vi "Shutter Control.vi"(8 "Laser Shutter":T1(radio)=enum."Off", 9 "error in":errorcluster, 11 "Camera Shutter":bool) -> ()   [LabVIEW 2014]
uses:
  Shutter SubVis/Global Shutter Variables - SubVI.vi
panel:
  out "error out":errorcluster
  out "Status":bool
  out "Current Wheel Position":string
  in  "Wheel Speed":u8=1 min=1 max=7 step=1
  in  "stop":bool
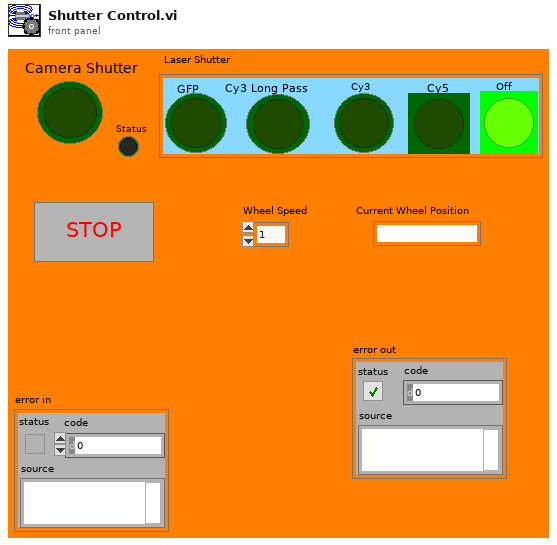
[diagram p1: front panel]
types:
  T1 = enum32{"No Selection", "GFP", "Cy3 Long Pass", "Cy3", "Cy5", "Off"}
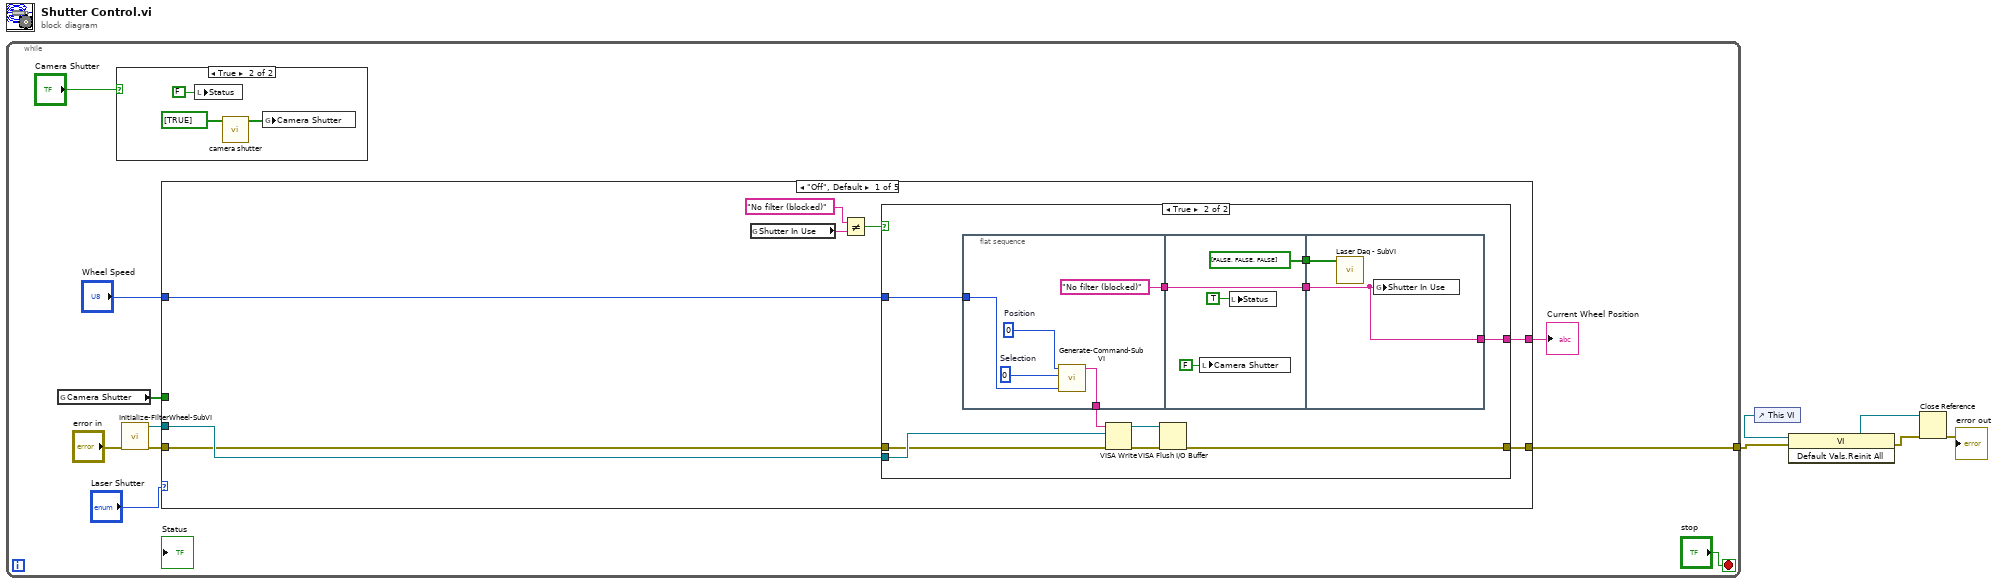
[diagram p0: block diagram]
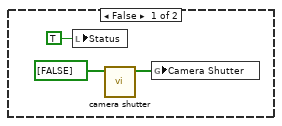
[diagram p2: hidden frame]
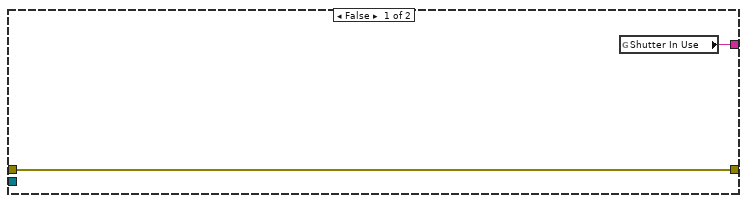
[diagram p3: hidden frame]
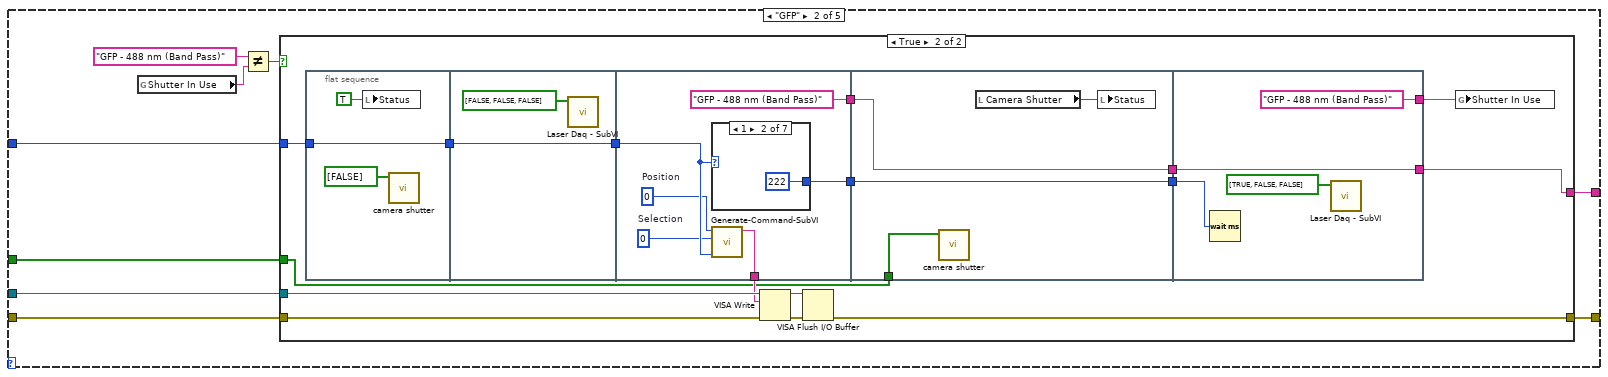
[diagram p4: hidden frame]
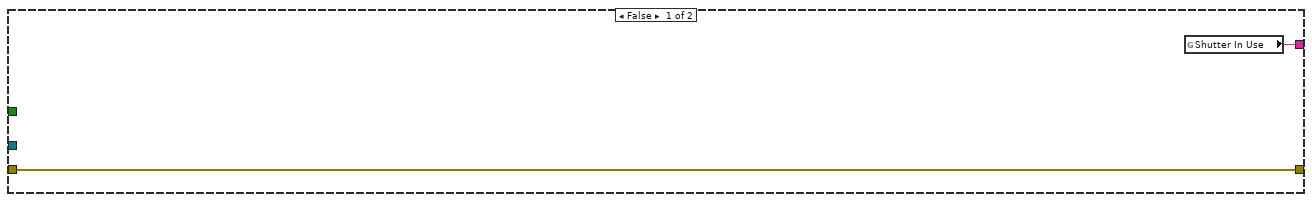
[diagram p5: hidden frame]
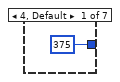
[diagram p6: hidden frame]
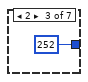
[diagram p7: hidden frame]
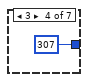
[diagram p8: hidden frame]
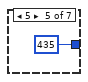
[diagram p9: hidden frame]
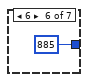
[diagram p10: hidden frame]
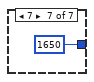
[diagram p11: hidden frame]
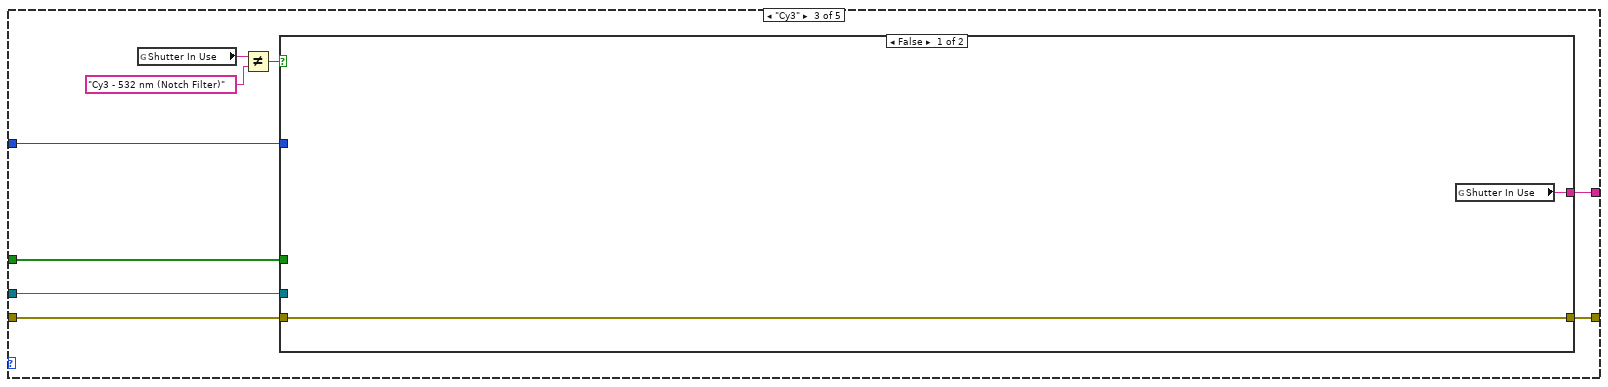
[diagram p12: hidden frame]
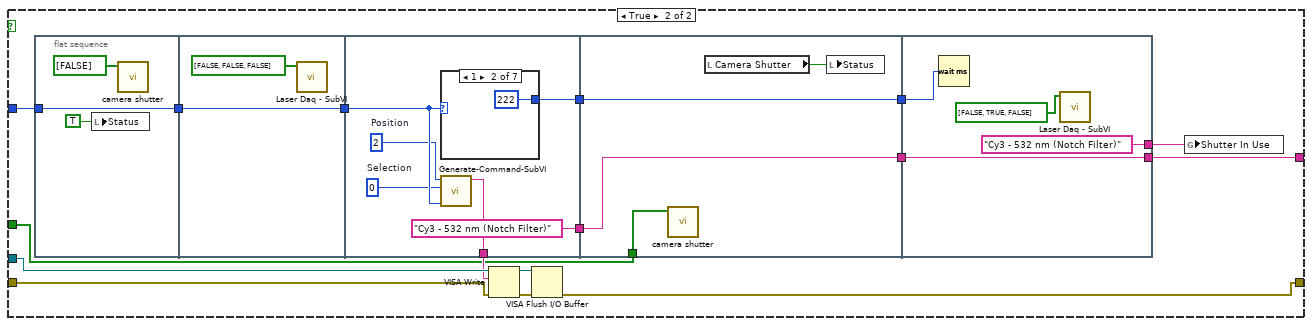
[diagram p13: hidden frame]
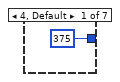
[diagram p14: hidden frame]
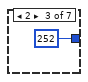
[diagram p15: hidden frame]
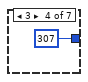
[diagram p16: hidden frame]
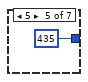
[diagram p17: hidden frame]
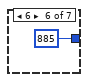
[diagram p18: hidden frame]
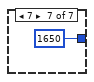
[diagram p19: hidden frame]
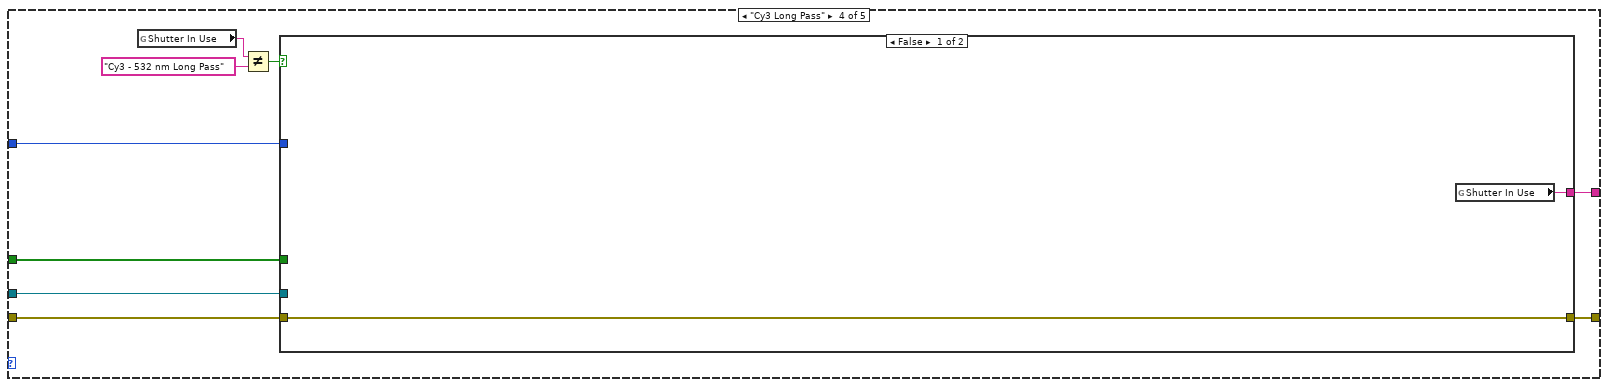
[diagram p20: hidden frame]
diagram:
  n1 = while {
    tunnel: [w6] -> w2
    stop <- "stop" stop-if-true
    n2 = global read "Global Shutter Variables - SubVI.vi" "Camera Shutter"() -> (w9:bool[])
    n3 = case shown="True" "Camera Shutter" {
      frame False {
        n4 = local write "Status"(TRUE ("Status")) -> ()
        n5 = call "camera shutter.vi"("Array"=bool[] [FALSE]) -> ("Array 2"=w17:bool[])  [unwired: 10 in]
        n6 = global write "Global Shutter Variables - SubVI.vi" "Camera Shutter"(w17) -> ()
      }
      frame True {
        n7 = local write "Status"(FALSE ("Status")) -> ()
        n8 = call "camera shutter.vi"("Array"=bool[] [TRUE]) -> ("Array 2"=w20:bool[])  [unwired: 10 in]
        n9 = global write "Global Shutter Variables - SubVI.vi" "Camera Shutter"(w20) -> ()
      }
    }
    n10 = call "Initialize-FilterWheel-SubVI.vi"("error in"="error in") -> ("VISA resource name out"=w12:refnum<visa-resource-name>, "error out"=w11:errorcluster)  [unwired: 8 in]
    n11 = case shown="\"Off\", Default" "Laser Shutter" {
      tunnel: "Wheel Speed" -> [w24 w62 w115 w168 w221]
      tunnel: w12 -> [w23 w61 w114 w167 w220]
      tunnel: w11 -> [w22 w55 w113 w166 w219]
      tunnel: [w26 w60 w112 w165 w218] -> w10
      tunnel: w9 -> [_ w56 w108 w161 w214]
      tunnel: [w25 w54 w107 w160 w213] -> w6
      frame "Off", Default {
        n12 = global read "Global Shutter Variables - SubVI.vi" "Shutter In Use"() -> (w28:string)
        n13 = Not Equal?(x="No filter (blocked)", y=w28) -> (x != y?=w29:bool)
        n14 = case shown="True" w29 {
          tunnel: [w31 w36] -> w26
          tunnel: [w30 w35] -> w25
          tunnel: w24 -> [_ w34]
          tunnel: w23 -> [_ w33]
          tunnel: w22 -> [w30 w32]
          frame False {
            n15 = global read "Global Shutter Variables - SubVI.vi" "Shutter In Use"() -> (w31:string)
          }
          frame True {
            n16 = flat-sequence {
              tunnel: [w45] -> w40
              tunnel: ["No filter (blocked)"] -> w38
              tunnel: w34 -> [w43]
              tunnel: [w50] -> w39
              tunnel: w38 -> [w50]
              tunnel: [bool[] [FALSE, FALSE, FALSE]] -> w37
              tunnel: w39 -> [w52]
              tunnel: w37 -> [w53]
              tunnel: [w52] -> w36
              frame #0 {
                w46 = 0  # Selection
                w47 = 0  # Position
                n17 = call "Generate-Command-SubVI.vi"("Wheel Speed"=w43, "Wheel Selection"=w46, "Wheel Position"=w47) -> ("type"=w45:string)  [unwired: 8 in]
              }
              frame #1 {
                n18 = local write "Camera Shutter"(FALSE ("Camera Shutter")) -> ()
                n19 = local write "Status"(TRUE ("Status")) -> ()
              }
              frame #2 {
                n20 = call "Laser Daq - SubVI.vi"("Array"=w53) -> ()  [unwired: 11 in]
                n21 = global write "Global Shutter Variables - SubVI.vi" "Shutter In Use"(w52) -> ()
              }
            }
            n22 = VISA Write(VISA resource name=w40, write buffer=w33, error in (no error)=w32) -> (VISA resource name out=w41:refnum<visa-resource-name>, error out=w42:errorcluster)  [unwired: 1 out]
            n23 = VISA Flush I/O Buffer(VISA resource name=w41, error in (no error)=w42) -> (error out=w35:errorcluster)  [unwired: 1 in, 1 out]
          }
        }
      }
      frame "GFP" {
        n24 = global read "Global Shutter Variables - SubVI.vi" "Shutter In Use"() -> (w58:string)
        n25 = Not Equal?(x="GFP - 488 nm (Band Pass)", y=w58) -> (x != y?=w57:bool)
        n26 = case shown="True" w57 {
          tunnel: w62 -> [_ w75]
          tunnel: w61 -> [_ w72]
          tunnel: w55 -> [w63 w71]
          tunnel: [w64 w69] -> w60
          tunnel: w56 -> [_ w66]
          tunnel: [w63 w65] -> w54
          frame False {
            n27 = global read "Global Shutter Variables - SubVI.vi" "Shutter In Use"() -> (w64:string)
          }
          frame True {
            n28 = flat-sequence {
              tunnel: w75 -> [w83]
              tunnel: [w83] -> w67
              tunnel: [w85] -> w80
              tunnel: w67 -> [w85]
              tunnel: [w88] -> w79
              tunnel: [w87] -> w70
              tunnel: ["GFP - 488 nm (Band Pass)"] -> w78
              tunnel: w80 -> [w91]
              tunnel: w79 -> [w101]
              tunnel: w78 -> [w102]
              tunnel: [w102] -> w77
              tunnel: [w101] -> w76
              tunnel: w66 -> [w100]
              tunnel: [w104] -> w69
              tunnel: w77 -> [w104]
              tunnel: w76 -> [w106]
              tunnel: ["GFP - 488 nm (Band Pass)"] -> w68
              frame #0 {
                n29 = local write "Status"(TRUE) -> ()
                n30 = call "camera shutter.vi"("Array"=bool[] [FALSE]) -> ()  [unwired: 10 in, 1 out]
              }
              frame #1 {
                n31 = call "Laser Daq - SubVI.vi"("Array"=bool[] [FALSE, FALSE, FALSE]) -> ()  [unwired: 11 in]
              }
              frame #2 {
                w89 = 0  # Selection
                w90 = 0  # Position
                n32 = case shown="1" w91 {
                  tunnel: [375 222 252 307 435 885 1650] -> w88
                  frame 4, Default {
                  }
                  frame 1 {
                  }
                  frame 2 {
                  }
                  frame 3 {
                  }
                  frame 5 {
                  }
                  frame 6 {
                  }
                  frame 7 {
                  }
                }
                n33 = call "Generate-Command-SubVI.vi"("Wheel Speed"=w91, "Wheel Selection"=w89, "Wheel Position"=w90) -> ("type"=w87:string)  [unwired: 8 in]
              }
              frame #3 {
                n34 = call "camera shutter.vi"("Array"=w100) -> ()  [unwired: 10 in, 1 out]
                n35 = local read "Camera Shutter"() -> (w99:bool)
                n36 = local write "Status"(w99) -> ()
              }
              frame #4 {
                n37 = Wait (ms)(milliseconds to wait=w106) -> ()  [unwired: 1 out]
                n38 = call "Laser Daq - SubVI.vi"("Array"=bool[] [TRUE, FALSE, FALSE]) -> ()  [unwired: 11 in]
              }
            }
            n39 = VISA Write(VISA resource name=w72, write buffer=w70, error in (no error)=w71) -> (VISA resource name out=w74:refnum<visa-resource-name>, error out=w73:errorcluster)  [unwired: 1 out]
            n40 = VISA Flush I/O Buffer(VISA resource name=w74, error in (no error)=w73) -> (error out=w65:errorcluster)  [unwired: 1 in, 1 out]
            n41 = global write "Global Shutter Variables - SubVI.vi" "Shutter In Use"(w68) -> ()
          }
        }
      }
      frame "Cy3" {
        n42 = global read "Global Shutter Variables - SubVI.vi" "Shutter In Use"() -> (w110:string)
        n43 = Not Equal?(x=w110, y="Cy3 - 532 nm (Notch Filter)") -> (x != y?=w109:bool)
        n44 = case shown="False" w109 {
          tunnel: w115 -> [_ w132]
          tunnel: w114 -> [_ w129]
          tunnel: w113 -> [w116 w128]
          tunnel: [w117 w126] -> w112
          tunnel: w108 -> [_ w119]
          tunnel: [w116 w118] -> w107
          frame False {
            n45 = global read "Global Shutter Variables - SubVI.vi" "Shutter In Use"() -> (w117:string)
          }
          frame True {
            n46 = flat-sequence {
              tunnel: w132 -> [w136]
              tunnel: [w136] -> w120
              tunnel: [w138] -> w133
              tunnel: w120 -> [w138]
              tunnel: [w141] -> w124
              tunnel: [w140] -> w127
              tunnel: ["Cy3 - 532 nm (Notch Filter)"] -> w122
              tunnel: w133 -> [w144]
              tunnel: w124 -> [w155]
              tunnel: [w155] -> w123
              tunnel: w122 -> [w154]
              tunnel: [w154] -> w121
              tunnel: w119 -> [w153]
              tunnel: w123 -> [w159]
              tunnel: [w158] -> w126
              tunnel: w121 -> [w158]
              tunnel: ["Cy3 - 532 nm (Notch Filter)"] -> w125
              frame #0 {
                n47 = local write "Status"(TRUE) -> ()
                n48 = call "camera shutter.vi"("Array"=bool[] [FALSE]) -> ()  [unwired: 10 in, 1 out]
              }
              frame #1 {
                n49 = call "Laser Daq - SubVI.vi"("Array"=bool[] [FALSE, FALSE, FALSE]) -> ()  [unwired: 11 in]
              }
              frame #2 {
                w142 = 0  # Selection
                w143 = 2  # Position
                n50 = case shown="1" w144 {
                  tunnel: [375 222 252 307 435 885 1650] -> w141
                  frame 4, Default {
                  }
                  frame 1 {
                  }
                  frame 2 {
                  }
                  frame 3 {
                  }
                  frame 5 {
                  }
                  frame 6 {
                  }
                  frame 7 {
                  }
                }
                n51 = call "Generate-Command-SubVI.vi"("Wheel Speed"=w144, "Wheel Selection"=w142, "Wheel Position"=w143) -> ("type"=w140:string)  [unwired: 8 in]
              }
              frame #3 {
                n52 = call "camera shutter.vi"("Array"=w153) -> ()  [unwired: 10 in, 1 out]
                n53 = local read "Camera Shutter"() -> (w152:bool)
                n54 = local write "Status"(w152) -> ()
              }
              frame #4 {
                n55 = Wait (ms)(milliseconds to wait=w159) -> ()  [unwired: 1 out]
                n56 = call "Laser Daq - SubVI.vi"("Array"=bool[] [FALSE, TRUE, FALSE]) -> ()  [unwired: 11 in]
              }
            }
            n57 = VISA Write(VISA resource name=w129, write buffer=w127, error in (no error)=w128) -> (VISA resource name out=w131:refnum<visa-resource-name>, error out=w130:errorcluster)  [unwired: 1 out]
            n58 = VISA Flush I/O Buffer(VISA resource name=w131, error in (no error)=w130) -> (error out=w118:errorcluster)  [unwired: 1 in, 1 out]
            n59 = global write "Global Shutter Variables - SubVI.vi" "Shutter In Use"(w125) -> ()
          }
        }
      }
      frame "Cy3 Long Pass" {
        n60 = global read "Global Shutter Variables - SubVI.vi" "Shutter In Use"() -> (w164:string)
        n61 = Not Equal?(x=w164, y="Cy3 - 532 nm Long Pass") -> (x != y?=w162:bool)
        n62 = case shown="False" w162 {
          tunnel: w168 -> [_ w185]
          tunnel: w167 -> [_ w182]
          tunnel: w166 -> [w169 w181]
          tunnel: [w170 w179] -> w165
          tunnel: w161 -> [_ w172]
          tunnel: [w169 w171] -> w160
          frame False {
            n63 = global read "Global Shutter Variables - SubVI.vi" "Shutter In Use"() -> (w170:string)
          }
          frame True {
            n64 = flat-sequence {
              tunnel: w185 -> [w189]
              tunnel: [w189] -> w177
              tunnel: [w191] -> w186
              tunnel: w177 -> [w191]
              tunnel: [w194] -> w176
              tunnel: [w193] -> w180
              tunnel: ["Cy3 - 532 nm Long Pass"] -> w174
              tunnel: w186 -> [w197]
              tunnel: w176 -> [w208]
              tunnel: [w208] -> w175
              tunnel: w174 -> [w207]
              tunnel: [w207] -> w173
              tunnel: w172 -> [w206]
              tunnel: w175 -> [w212]
              tunnel: [w211] -> w179
              tunnel: w173 -> [w211]
              tunnel: ["Cy3 - 532 nm Long Pass"] -> w178
              frame #0 {
                n65 = local write "Status"(TRUE) -> ()
                n66 = call "camera shutter.vi"("Array"=bool[] [FALSE]) -> ()  [unwired: 10 in, 1 out]
              }
              frame #1 {
                n67 = call "Laser Daq - SubVI.vi"("Array"=bool[] [FALSE, FALSE, FALSE]) -> ()  [unwired: 11 in]
              }
              frame #2 {
                w195 = 0  # Selection
                w196 = 5  # Position
                n68 = case shown="7" w197 {
                  tunnel: [375 222 252 307 435 885 1650] -> w194
                  frame 4, Default {
                  }
                  frame 1 {
                  }
                  frame 2 {
                  }
                  frame 3 {
                  }
                  frame 5 {
                  }
                  frame 6 {
                  }
                  frame 7 {
                  }
                }
                n69 = call "Generate-Command-SubVI.vi"("Wheel Speed"=w197, "Wheel Selection"=w195, "Wheel Position"=w196) -> ("type"=w193:string)  [unwired: 8 in]
              }
              frame #3 {
                n70 = call "camera shutter.vi"("Array"=w206) -> ()  [unwired: 10 in, 1 out]
                n71 = local read "Camera Shutter"() -> (w205:bool)
                n72 = local write "Status"(w205) -> ()
              }
              frame #4 {
                n73 = Wait (ms)(milliseconds to wait=w212) -> ()  [unwired: 1 out]
                n74 = call "Laser Daq - SubVI.vi"("Array"=bool[] [FALSE, TRUE, FALSE]) -> ()  [unwired: 11 in]
              }
            }
            n75 = VISA Write(VISA resource name=w182, write buffer=w180, error in (no error)=w181) -> (VISA resource name out=w184:refnum<visa-resource-name>, error out=w183:errorcluster)  [unwired: 1 out]
            n76 = VISA Flush I/O Buffer(VISA resource name=w184, error in (no error)=w183) -> (error out=w171:errorcluster)  [unwired: 1 in, 1 out]
            n77 = global write "Global Shutter Variables - SubVI.vi" "Shutter In Use"(w178) -> ()
          }
        }
      }
      frame "Cy5" {
        n78 = global read "Global Shutter Variables - SubVI.vi" "Shutter In Use"() -> (w217:string)
        n79 = Not Equal?(x=w217, y="Cy5 - 637 (Notch Filter)") -> (x != y?=w215:bool)
        n80 = case shown="False" w215 {
          tunnel: w221 -> [_ w238]
          tunnel: w220 -> [_ w235]
          tunnel: w219 -> [w222 w234]
          tunnel: [w223 w232] -> w218
          tunnel: w214 -> [_ w225]
          tunnel: [w222 w224] -> w213
          frame False {
            n81 = global read "Global Shutter Variables - SubVI.vi" "Shutter In Use"() -> (w223:string)
          }
          frame True {
            n82 = flat-sequence {
              tunnel: w238 -> [w242]
              tunnel: [w242] -> w230
              tunnel: [w244] -> w239
              tunnel: w230 -> [w244]
              tunnel: [w247] -> w229
              tunnel: [w246] -> w233
              tunnel: ["Cy5 - 637 (Notch Filter)"] -> w227
              tunnel: w239 -> [w250]
              tunnel: w229 -> [w261]
              tunnel: [w261] -> w228
              tunnel: w227 -> [w260]
              tunnel: [w260] -> w226
              tunnel: w225 -> [w259]
              tunnel: w228 -> [w265]
              tunnel: [w264] -> w232
              tunnel: w226 -> [w264]
              tunnel: ["Cy5 - 637 (Notch Filter)"] -> w231
              frame #0 {
                n83 = local write "Status"(TRUE) -> ()
                n84 = call "camera shutter.vi"("Array"=bool[] [FALSE]) -> ()  [unwired: 10 in, 1 out]
              }
              frame #1 {
                n85 = call "Laser Daq - SubVI.vi"("Array"=bool[] [FALSE, FALSE, FALSE]) -> ()  [unwired: 11 in]
              }
              frame #2 {
                w248 = 0  # Selection
                w249 = 7  # Position
                n86 = case shown="1" w250 {
                  tunnel: [375 222 252 307 435 885 1650] -> w247
                  frame 4, Default {
                  }
                  frame 1 {
                  }
                  frame 2 {
                  }
                  frame 3 {
                  }
                  frame 5 {
                  }
                  frame 6 {
                  }
                  frame 7 {
                  }
                }
                n87 = call "Generate-Command-SubVI.vi"("Wheel Speed"=w250, "Wheel Selection"=w248, "Wheel Position"=w249) -> ("type"=w246:string)  [unwired: 8 in]
              }
              frame #3 {
                n88 = call "camera shutter.vi"("Array"=w259) -> ()  [unwired: 10 in, 1 out]
                n89 = local read "Camera Shutter"() -> (w258:bool)
                n90 = local write "Status"(w258) -> ()
              }
              frame #4 {
                n91 = Wait (ms)(milliseconds to wait=w265) -> ()  [unwired: 1 out]
                n92 = call "Laser Daq - SubVI.vi"("Array"=bool[] [FALSE, FALSE, TRUE]) -> ()  [unwired: 11 in]
              }
            }
            n93 = VISA Write(VISA resource name=w235, write buffer=w233, error in (no error)=w234) -> (VISA resource name out=w237:refnum<visa-resource-name>, error out=w236:errorcluster)  [unwired: 1 out]
            n94 = VISA Flush I/O Buffer(VISA resource name=w237, error in (no error)=w236) -> (error out=w224:errorcluster)  [unwired: 1 in, 1 out]
            n95 = global write "Global Shutter Variables - SubVI.vi" "Shutter In Use"(w231) -> ()
          }
        }
      }
    }
    "Current Wheel Position" <- w10
  }
  n96 = control-ref of="This VI"() -> (w5:refnum<vi>)
  n97 = invoke class="VI" method="Default Vals.Reinit All"(reference=w5, error in=w2) -> (reference out=w3:refnum<vi>, error out=w4:errorcluster)  [unwired: 1 in, 1 out]
  n98 = Close Reference(reference=w3, error in (no error)=w4) -> (error out=→"error out":errorcluster)
